vi "ConfigDO.vi"(0 "object in":refnum<class "AD2_SDK.lvclass">, 2 "?":T1={"DO Trigger"={"secRun(0=Cont)"=0.0, "secWait"=0.0, "cRepeat(0=inf)"=0, "Repeat Trigger"=FALSE, "TrigrSrc"=enum."trigrsrcNone"}, "CustomData"=[{"Data"=[FALSE, TRUE, FALSE, FALSE, FALSE, FALSE, FALSE, FALSE, FALSE, FALSE, FALSE, FALSE, FALSE, FALSE, FALSE, FALSE, FALSE, FALSE, FALSE, FALSE, FALSE, FALSE], "Freq"=1000.0, "#Bits"=100, "Enable"=FALSE}, {"Data"=[TRUE, TRUE, TRUE, TRUE, TRUE, FALSE, FALSE, FALSE, FALSE, FALSE, FALSE, FALSE, FALSE, FALSE, FALSE, FALSE, FALSE, FALSE, FALSE, FALSE, FALSE, FALSE], "Freq"=1000.0, "#Bits"=100, "Enable"=FALSE}, {"Data"=[], "Freq"=0.0, "#Bits"=0, "Enable"=FALSE}, {"Data"=[FALSE, FALSE, FALSE, FALSE, FALSE, FALSE, FALSE, FALSE, FALSE, FALSE, FALSE, FALSE, FALSE, FALSE, FALSE, FALSE, FALSE, FALSE, FALSE, FALSE, FALSE, FALSE, FALSE], "Freq"=0.0, "#Bits"=0, "Enable"=FALSE}, {"Data"=[], "Freq"=0.0, "#Bits"=0, "Enable"=FALSE}, {"Data"=[], "Freq"=0.0, "#Bits"=0, "Enable"=FALSE}, {"Data"=[], "Freq"=0.0, "#Bits"=0, "Enable"=FALSE}, {"Data"=[], "Freq"=0.0, "#Bits"=0, "Enable"=FALSE}, {"Data"=[], "Freq"=0.0, "#Bits"=0, "Enable"=FALSE}, {"Data"=[], "Freq"=0.0, "#Bits"=0, "Enable"=FALSE}, {"Data"=[], "Freq"=0.0, "#Bits"=0, "Enable"=FALSE}, {"Data"=[], "Freq"=0.0, "#Bits"=0, "Enable"=FALSE}, {"Data"=[], "Freq"=0.0, "#Bits"=0, "Enable"=FALSE}, {"Data"=[], "Freq"=0.0, "#Bits"=0, "Enable"=FALSE}, {"Data"=[], "Freq"=0.0, "#Bits"=0, "Enable"=FALSE}, {"Data"=[FALSE, FALSE, FALSE, FALSE, FALSE, FALSE, FALSE, FALSE, FALSE, FALSE, FALSE, FALSE, FALSE, FALSE, FALSE, FALSE, FALSE, FALSE, FALSE, FALSE, FALSE, FALSE, FALSE], "Freq"=0.0, "#Bits"=0, "Enable"=FALSE}, {"Data"=[FALSE, FALSE, FALSE, FALSE, FALSE, FALSE, FALSE, FALSE, FALSE, FALSE, FALSE, FALSE, FALSE, FALSE, FALSE, FALSE, FALSE, FALSE, FALSE, FALSE, FALSE, FALSE, FALSE], "Freq"=0.0, "#Bits"=0, "Enable"=FALSE}]}, 5 "error in (no error)":errorcluster) -> (14 "object out":refnum<class "AD2_SDK.lvclass">, 19 "error out":errorcluster)   [LabVIEW 2021, in "AD2_SDK.lvclass"]
uses:
  AD2_SDK.lvclass
  AD2_SDK.lvclass/AD2_SDK.ctl
  AD2_DO_SDK_class/AD2_DO_SDK.lvclass
  AD2_DO_SDK_class/DOCustomData.ctl
  AD2_WFG_SDK_class/AD2TriggerSources.ctl
  AD2_DO_SDK_class/DOTrigger.ctl
  AD2_DO_SDK_class/DOConfigureCustomData.ctl
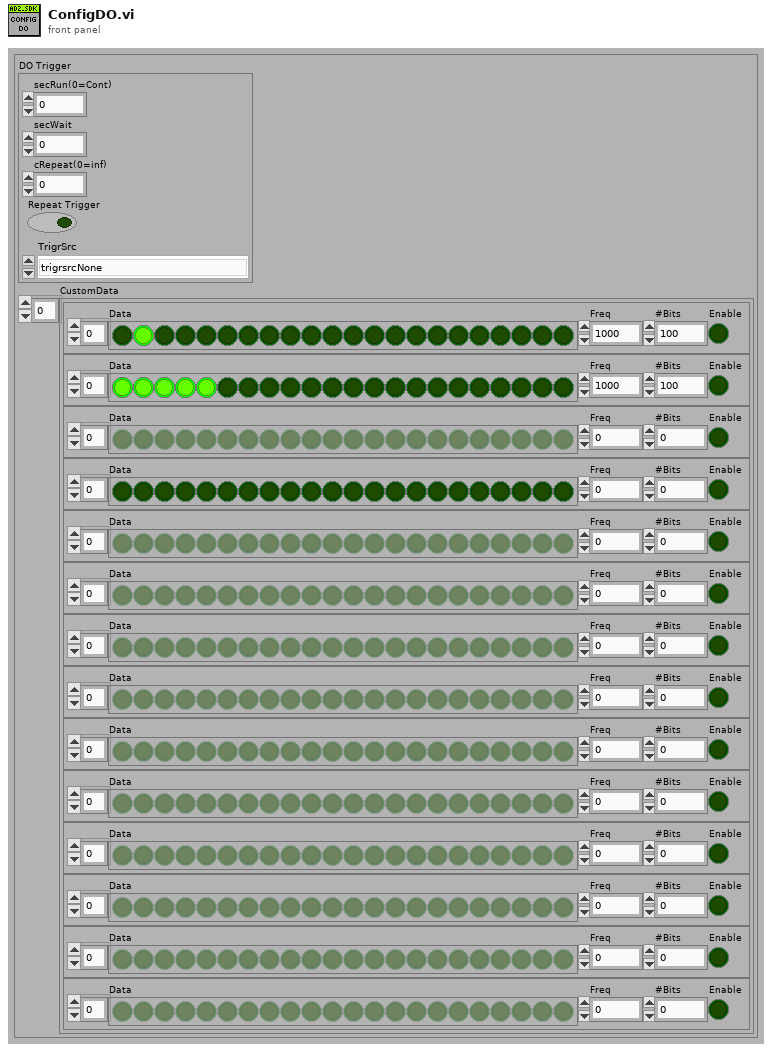
[diagram p1: front panel]
types:
  T1 = typedef "DOConfigureCustomData.ctl" = cluster{"DO Trigger":T2, "CustomData":T4}
  T2 = typedef "AD2_DO_SDK.lvclass/DOTrigger.ctl" = cluster{"secRun(0=Cont)":dbl, "secWait":dbl, "cRepeat(0=inf)":i32, "Repeat Trigger":bool, "TrigrSrc":T3}
  T3 = typedef "AD2_SDK.lvclass/AD2TriggerSources.ctl" = enum8{"trigrsrcNone", "trigsrcPC", "trigsrcDetectorAnalogIn", "trigsrcDetectorDigitalIn", "trigsrcAnalogIn", "trigsrcDigitalIn", "trigsrcDigitalOut", "trigsrcAnalogOut1", "trigsrcAnalogOut2", "trigsrcAnalogOut3", "trigsrcAnalogOut4", "trigsrcExternal1", "trigsrcExternal2", "trigsrcExternal3", "trigsrcExternal4", ""}
  T4 = typedef "AD2_DO_SDK.lvclass/DOCustomData.ctl" = cluster{"Data":bool[], "Freq":dbl, "#Bits":u32, "Enable":bool}[]
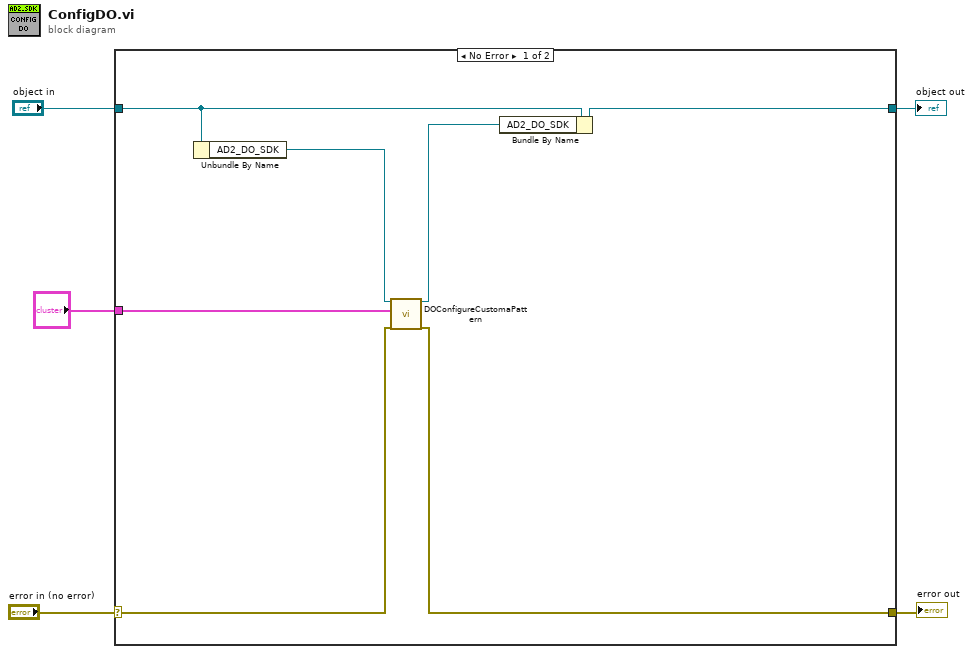
[diagram p0: block diagram]
diagram:
  n1 = case shown="No Error" "error in (no error)" {
    selector: "error in (no error)" -> [w7 w14]
    tunnel: [w6 w14] -> w4
    tunnel: [w9 w13] -> w2
    tunnel: "object in" -> [w12 w13]
    tunnel: "?" -> [w11 _]
    frame No Error {
      n2 = Unbundle By Name(w12) -> ("AD2_DO_SDK"=w10:refnum<class "AD2_DO_SDK.lvclass">)
      n3 = call-dynamic "DOConfigureCustomaPattern.vi"("object in"=w10, 2:w11, "error in (no error)"=w7) -> ("object out"=w8:refnum<class "AD2_DO_SDK.lvclass">, "error out"=w6:errorcluster)  [unwired: 15 in]
      n4 = Bundle By Name(cluster=w12, "AD2_DO_SDK"=w8) -> (w9:refnum<class "AD2_SDK.lvclass">)
    }
    frame Error {
    }
  }
  "error out" <- w4
  "object out" <- w2
